vi "main 0.1.vi"() -> ()   [LabVIEW 2015]
uses:
  subvi/Newport ESP301/Newport ESP301.lvlib
  subvi/sp_manip.llb/sp_manip_lib.lvlib
  subvi/sp_manip.llb/tcp_gateway.lvlib
panel:
  out "error IO":errorcluster
  out "ESP_con?":bool caption="ESP301"
  out "phoib_con?":bool caption="PHOIBOS"
  out "manip_con?":bool caption="manipulator"
  out "cam_con?":bool caption="camera"
  in  "main_close":bool
  in  "Tab Control":enum32{"Live", "Measure", "Settings", "Devices"}(tab)
  out "Intensity Graph":u16[][](graph)
  out "Saved Positions":string[][](table)=[["ertwertwert", "-2.299945", "-2.030214", "38.900024", "50.000762", "0.000887", "-97.998082"], ["uztgugt", "-14.999451", "-13.638894", "442.380066", "13.998380", "-1.893758", "-76.305838"], ["asdf", "-14.999451", "-13.638894", "442.380066", "13.998380", "-1.893758", "-76.305838"], ["test3", "-14.999451", "-13.638894", "441.380066", "13.998380", "-1.893758", "-76.305838"]]
  in  "Save Pos":bool
  in  "Load":bool
  in  "Delete":bool
  in  "ManipRel":dbl=1.0
  in  "ManipRel +":bool
  in  "ManipRel -":bool
  in  "manip.rel.select":enum32{"x", "y", "z", "polar", "tilt", "azimut"}(radio)=enum."polar"
  in  "Move Abs":bool
  in  "stop manip":bool
  in  "dest":dbl[](array[numeric])=[0.007141549166819264, -0.009888298846365134, 431.30615234375, 89.00040512814502, 1.109125024699864, -227.9162918846475] caption="destinations" format="%#.5g"
  out "names":string[](array[string])=["x", "y", "z", "polar", "tilt", "azimut"]
  out "pos":dbl[](array[numeric])=[0.007141549166819264, -0.009888298846365134, 431.30615234375, 89.00040512814502, 1.109125024699864, -227.9162918846475] caption="positions" format="%.5f"
  in  "Delay":dbl format="%.1f"
  in  "Exposure":dbl=1000.0 format="%.1f"
  in  "Vertical binning":u16=4
  in  "Horzontal binning":u16=4
  in  "ROI Bottom":i32=33
  in  "ROI Top":i32=1
  in  "ROI Right":i32=43
  in  "ROI Left":i32=1
  out "opti_frames":dbl=25.0 caption="#steps_opti"
  out "opti_current_frame":i32=25
  out "Measurement Progress":u8(slide) scale=0.0..100.0
  out "Camera Aquisition":u8(slide) scale=0.0..100.0
  in  "Optimize":bool
  in  "OptiStepSize":dbl=-1.0 caption="Step Size"
  in  "OptiRange":dbl=25.0 caption="Range"
  in  "meas_axis":string(combo)="tilt" caption="Axis"
  in  "OptiFrameAcc.":i32=60 caption="Frames2Average"
  in  "OptiCancel":bool
  out "#steps_opti":dbl=25.0
  out "current_step_opti":i32=25
  out "ETA":string
  in  "BasePath":path=path "Z:/PESdata"
  in  "Path":path=path "Z:/software/ManipulatorControl/save.txt"
  in  "ESP301 VISA":refnum<visa-resource-name>
  in  "cam_boardnr":i32
  # "step _ of _"
  # "step _ of _"
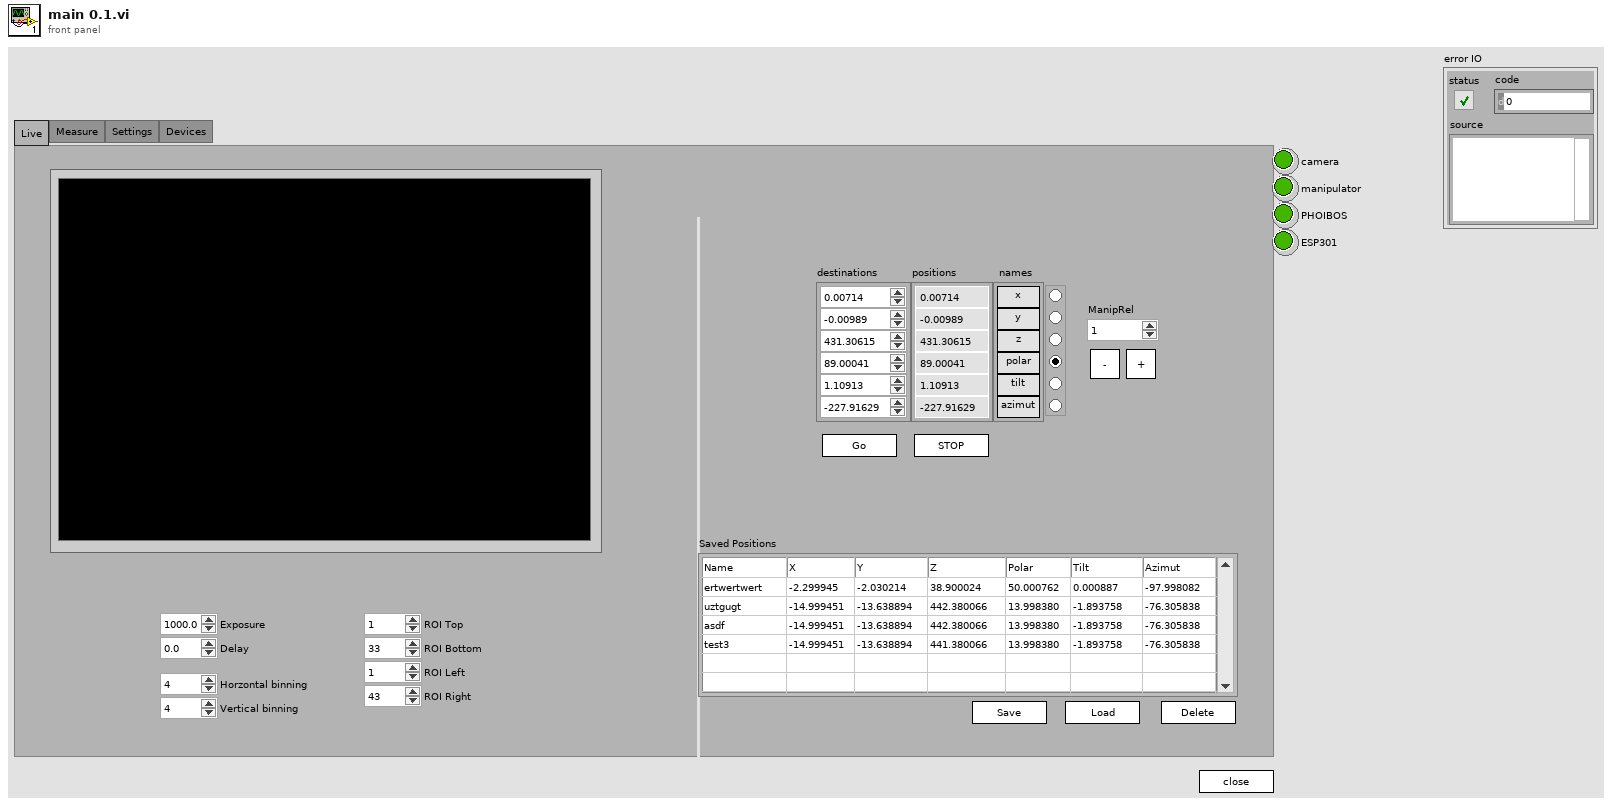
[diagram p1: front panel]
types:
  T1 = cluster{"Camera type":u32, "Operating mode\nHP & QE / HS & DiCam Pro ":u32, "Frame trigger \n(High Performance and QE only)":u16, "Sequence trigger":u16, "Low Light\n(QE only)":bool, "Gain":bool, "Horzontal\nbinning":u16, "Vertical\nbinning ":u16, "ROI Left":i32, "ROI Right":i32, "ROI Top":i32, "ROI Bottom":i32}
  T2 = cluster{"Axis_Name":string, "Axis_Type":string, "Axis_Position":dbl, "continous":bool, "moving":bool}[]
  T3 = cluster{"Axis_Name":string, "Axis_Type":string, "Axis_Position":dbl, "continous":bool, "moving":bool}
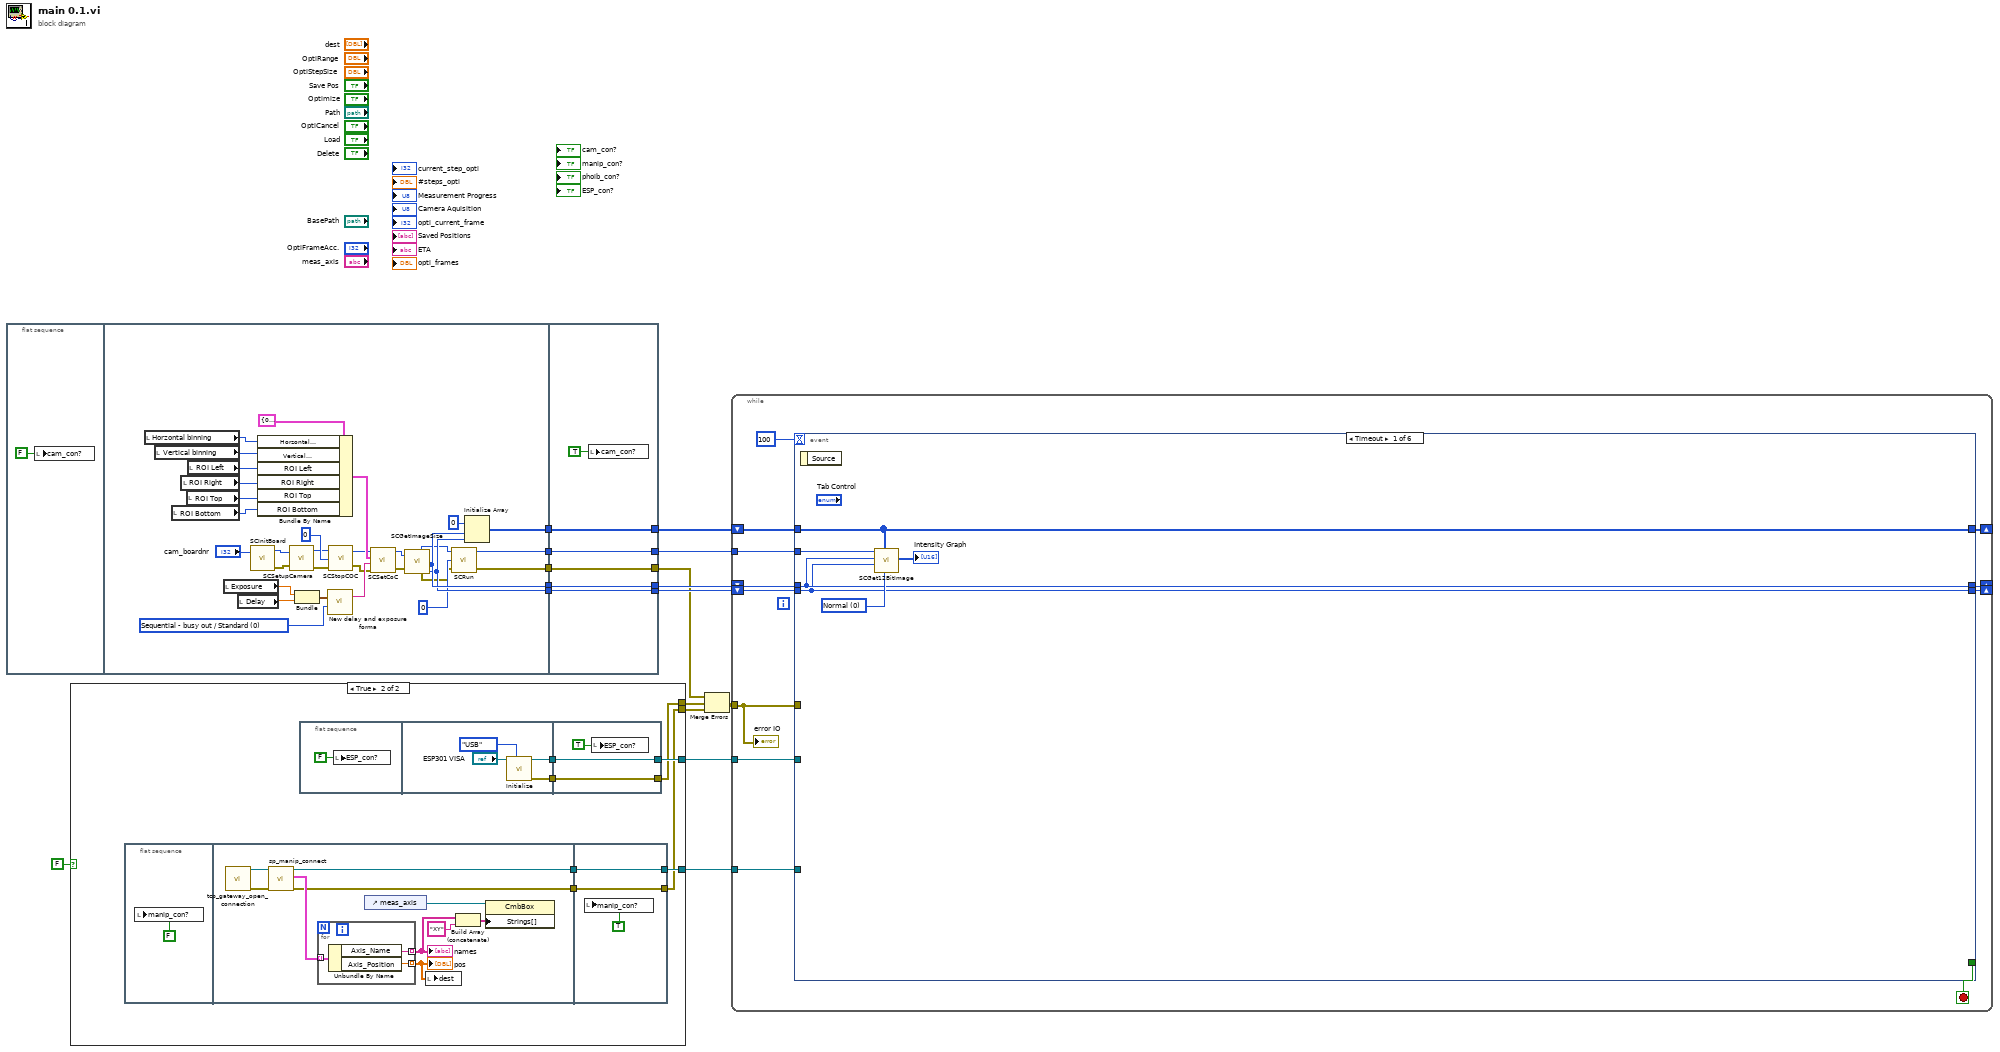
[diagram p0: block diagram]
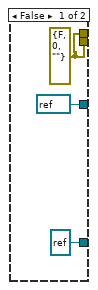
[diagram p2: hidden frame]
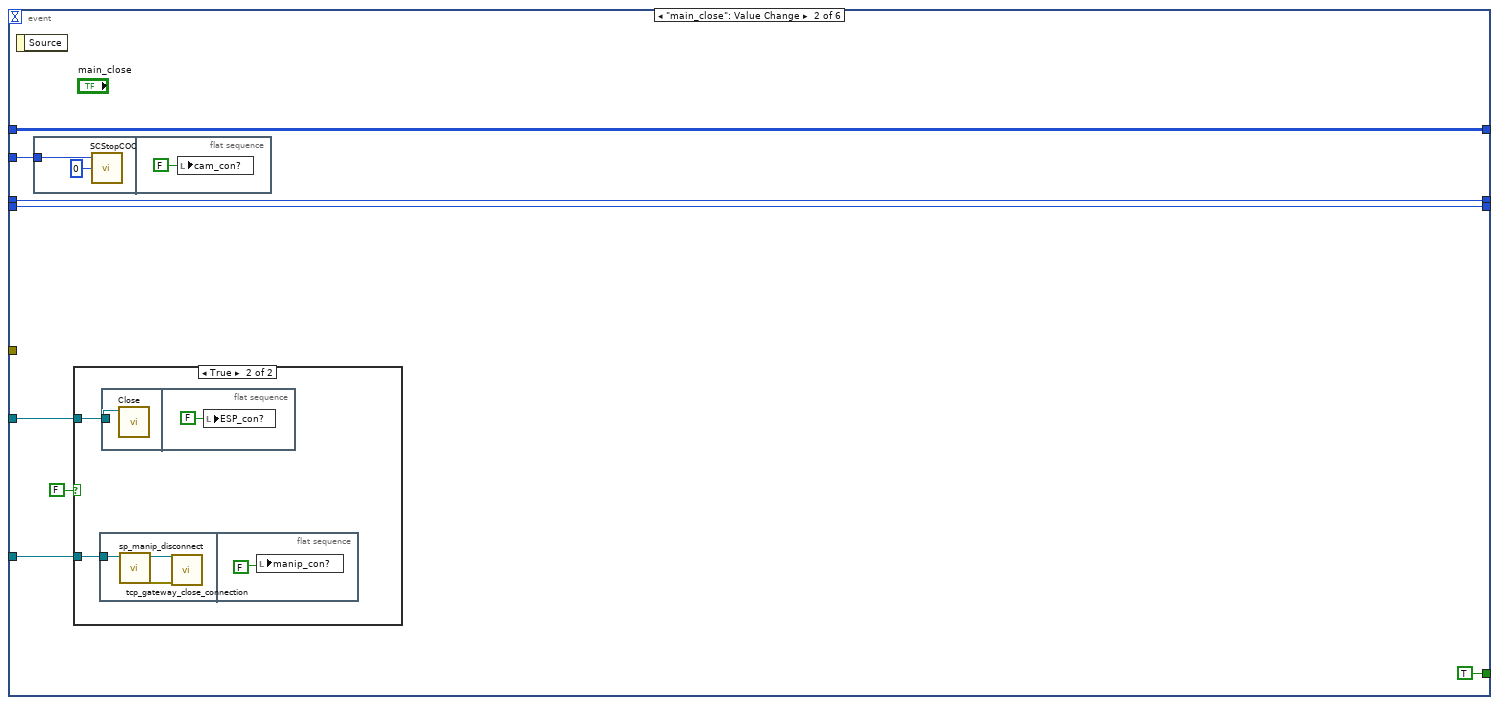
[diagram p3: hidden frame]
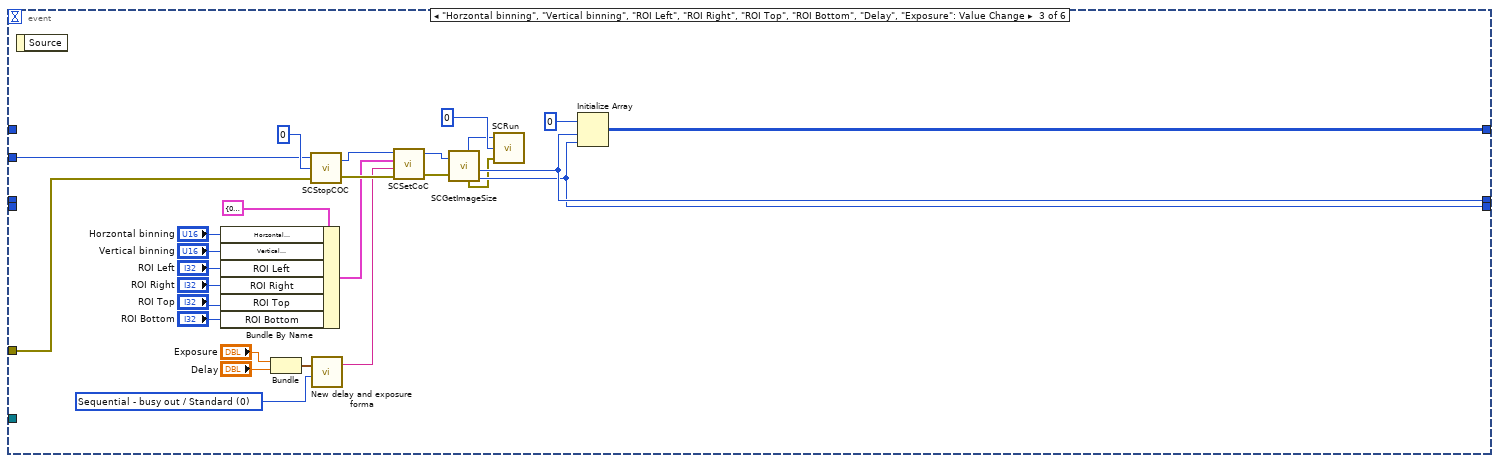
[diagram p5: hidden frame]
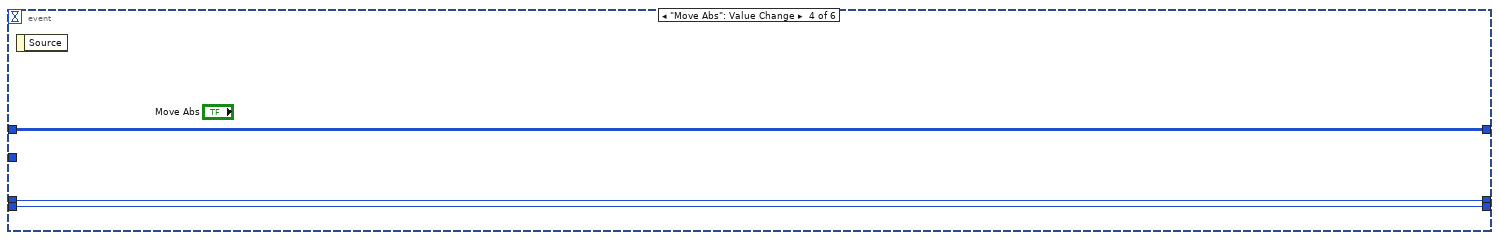
[diagram p6: hidden frame]
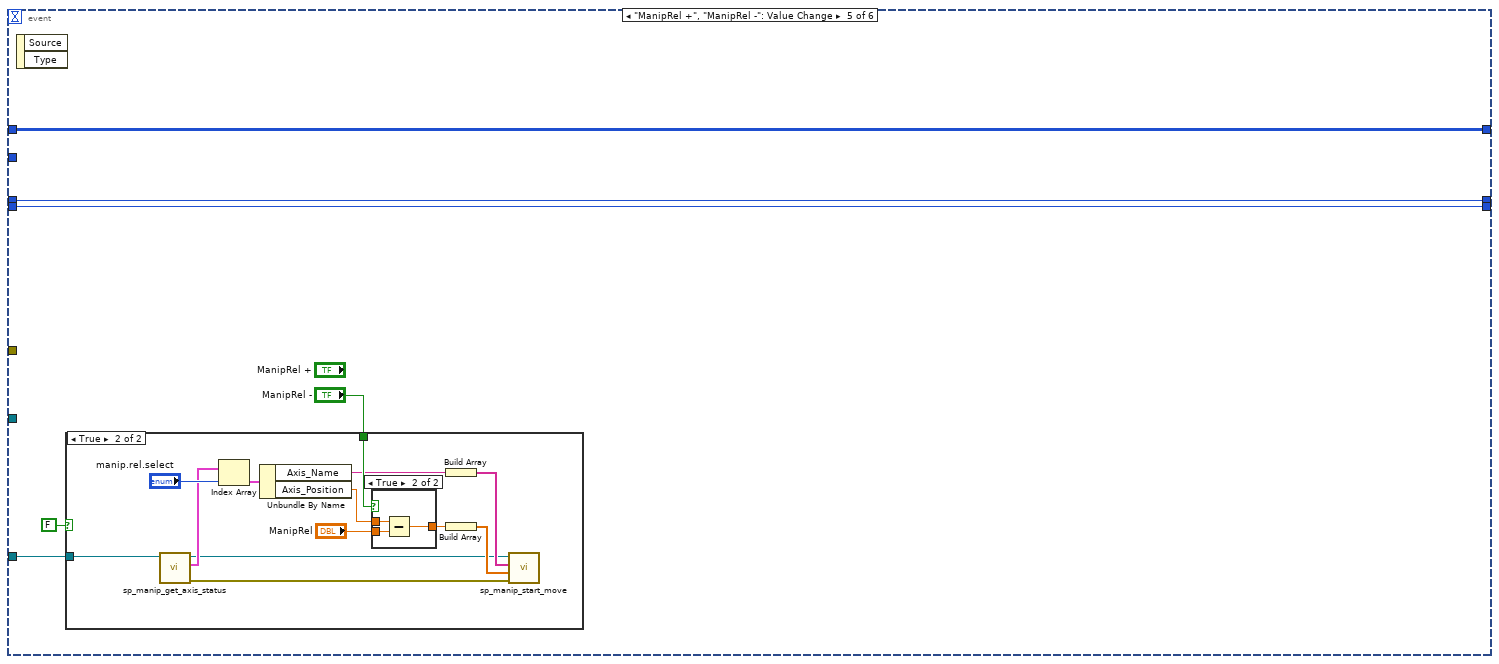
[diagram p7: hidden frame]
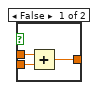
[diagram p9: hidden frame]
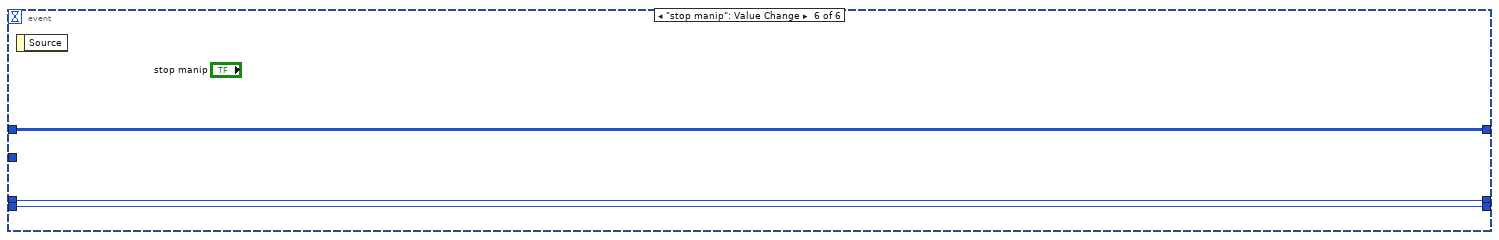
[diagram p10: hidden frame]
diagram:
  n1 = flat-sequence {
    tunnel: [w42] -> w6
    tunnel: [w38] -> w5
    tunnel: [w37] -> w4
    tunnel: [w28] -> w3
    tunnel: [w27] -> w2
    tunnel: [w51] -> w7
    tunnel: [w52] -> w8
    tunnel: [w53] -> w9
    tunnel: [w54] -> w10
    tunnel: [w55] -> w11
    tunnel: w6 -> [w55]
    tunnel: w5 -> [w54]
    tunnel: w4 -> [w53]
    tunnel: w3 -> [w52]
    tunnel: w2 -> [w51]
    frame #0 {
      n2 = local write "cam_con?"(FALSE ("cam_con?")) -> ()
    }
    frame #1 {
      w26 = u32 0 items=["Sequential - busy out / Standard"=0, "Simultaneous - busy out / 200 ns Double shot"=1, "Sequential - exposure out / 1000 ns Double shot"=2, "Simultaneous - exposure out / Reserved"=3, "Fast Frame / Fast cycle"=5, "QE short exposure"=8, "QE double shot"=9] ("Operating mode\nHP & QE / HS & DiCam Pro")
      n3 = local read "Horzontal binning"() -> (w36:u16)
      n4 = local read "Vertical binning"() -> (w35:u16)
      n5 = local read "ROI Bottom"() -> (w31:i32)
      n6 = local read "ROI Right"() -> (w33:i32)
      n7 = local read "ROI Top"() -> (w32:i32)
      n8 = local read "ROI Left"() -> (w34:i32)
      n9 = local read "Exposure"() -> (w25:dbl)
      n10 = local read "Delay"() -> (w24:dbl)
      n11 = call "SCInitBoard.vi"("boardnr"="cam_boardnr") -> ("Hout"=w47:u32, "error out"=w46:errorcluster)  [unwired: 1 in, 1 out]
      n12 = Bundle By Name(cluster=T1 {"Camera type"=0, "Operating mode\nHP & QE / HS & DiCam Pro "=0, "Frame trigger \n(High Performance and QE only)"=0, "Sequence trigger"=0, "Low Light\n(QE only)"=FALSE, "Gain"=FALSE, "Horzontal\nbinning"=0, "Vertical\nbinning "=0, "ROI Left"=1, "ROI Right"=20, "ROI Top"=1, "ROI Bottom"=15} ("Camera controls"), "Horzontal\nbinning"=w36, "Vertical\nbinning"=w35, "ROI Left"=w34, "ROI Right"=w33, "ROI Top"=w32, "ROI Bottom"=w31) -> (w40:T1)
      n13 = call "SCSetupCamera.vi"("Handle"=w47, "error in (no error)"=w46) -> ("Hout"=w45:u64, "error out"=w44:errorcluster)  [unwired: 1 out]
      n14 = Bundle("Exposure"=w25, "Delay"=w24) -> (w39:cluster{"Exposure ":dbl, "Delay":dbl})  [unwired: 1 in]
      n15 = call "New delay and exposure forma.vi"("Operating mode\nHP & QE / HS & DiCam Pro"=w26, "Delay and exposure"=w39) -> ("Output table"=w30:string)  [unwired: 3 in]
      n16 = call "SCStopCOC.vi"("error in (no error)"=w44, "Stop mode"=0, "Handle"=w45) -> ("error out"=w23:errorcluster, "Hout"=w22:u64)
      n17 = call "SCSetCoC.vi"("error in (no error)"=w23, "Delay and exposure table"=w30, "Camera controls"=w40, "Handle"=w22) -> ("error out"=w20:errorcluster, "Hout"=w21:u64)  [unwired: 1 out]
      n18 = call "SCGetImageSize.vi"("Handle"=w21, "error in (no error)"=w20) -> ("Hout"=w19:u64, "error out"=w18:errorcluster, "Horizontal size"=w38:i32, "Vertical size"=w37:i32)  [unwired: 2 out]
      n19 = call "SCRun.vi"("error in (no error)"=w18, "Run mode"=0, "Handle"=w19) -> ("error out"=w27:errorcluster, "Run error out"=w28:i32)  [unwired: 1 out]
      n20 = Initialize Array(u16 0 ("dimension size"), w38, w37) -> (w42:u16[][])
    }
    frame #2 {
      n21 = local write "cam_con?"(TRUE ("cam_con?")) -> ()
    }
  }
  n22 = case shown="True" FALSE {
    tunnel: [refnum<visa-resource-name> refnum ("VISA resource name out") w62] -> w16
    tunnel: [refnum<k5> refnum ("gateway_connection out") w61] -> w15
    tunnel: [w56 w60] -> w14
    tunnel: [w56 w59] -> w13
    frame False {
      w56 = errorcluster {"status"=FALSE, "code"=0, "source"=""} ("error out")
    }
    frame True {
      n23 = flat-sequence {
        tunnel: [w77] -> w66
        tunnel: [w85] -> w65
        tunnel: [w90] -> w61
        tunnel: [w91] -> w60
        tunnel: w66 -> [w91]
        tunnel: w65 -> [w90]
        frame #0 {
          n24 = local write "manip_con?"(FALSE ("manip_con?")) -> ()
        }
        frame #1 {
          n25 = call "tcp_gateway_open_connection.vi"() -> ("gateway_connection"=w80:refnum<k5>, "error out"=w79:errorcluster)  [unwired: 5 in, 3 out]
          n26 = call "sp_manip_connect.vi"("error in"=w79, "gateway_connection"=w80) -> ("error out"=w77:errorcluster, "axis_out"=w78:T2, "gateway_connection out"=w85:refnum<k5>)  [unwired: 5 in, 2 out]
          n27 = for {
            tunnel: w78 -> [w88] mode=indexing
            tunnel: [w87] -> w83 mode=indexing
            tunnel: [w86] -> w84 mode=indexing
            n28 = Unbundle By Name(w88) -> ("Axis_Name"=w87:string, "Axis_Position"=w86:dbl)
          }
          "names" <- w83
          "pos" <- w84
          n29 = control-ref of="meas_axis"() -> (w76:refnum<vi>)
          n30 = local write "dest"(w84) -> ()
          n31 = Build Array (concatenate)(w83, "XY") -> (w81:string[])
          n32 = property on="Property Node" class="CmbBox"(reference=w76, "Strings[]"=w81) -> ()  [unwired: 1 in, 2 out]
        }
        frame #2 {
          n33 = local write "manip_con?"(TRUE ("manip_con?")) -> ()
        }
      }
      n34 = flat-sequence {
        tunnel: [w69] -> w64
        tunnel: [w68] -> w63
        tunnel: [w73] -> w59
        tunnel: [w74] -> w62
        tunnel: w64 -> [w74]
        tunnel: w63 -> [w73]
        frame #0 {
          n35 = local write "ESP_con?"(FALSE ("manip_con?")) -> ()
        }
        frame #1 {
          n36 = call "Initialize.vi"("VISA resource name"="ESP301 VISA", "Serial Link (RS232)"=enum16{"RS232", "USB"}."USB") -> ("VISA resource name out"=w69:refnum<visa-resource-name>, "error out"=w68:errorcluster)  [unwired: 7 in]
        }
        frame #2 {
          n37 = local write "ESP_con?"(TRUE ("manip_con?")) -> ()
        }
      }
    }
  }
  n38 = Merge Errors(w7, w13, w14) -> (w12:errorcluster)
  n39 = while {
    tunnel: w16 -> [w102]
    tunnel: w12 -> [w101]
    tunnel: w15 -> [w100]
    tunnel: w8 -> [w98]
    shift-right: [w94] -> _
    shift-left: w10 -> [w97]
    shift-right: [w93] -> _
    shift-left: w9 -> [w96]
    shift-right: [w92] -> _
    shift-left: w11 -> [w99]
    stop <- w103 stop-if-true
    n40 = event shown="[0] Timeout" {
      selector: _ -> [_ _ _ _ _ _]
      dyn-events: _ -> [_ _ _ _ _ _]
      timeout: 100 -> [_ _ _ _ _ _]
      tunnel: [_ TRUE _ _ _ _] -> w103
      tunnel: w102 -> [_ w116 _ _ _ _]
      tunnel: w101 -> [_ _ w137 _ _ _]
      tunnel: w100 -> [_ w115 _ _ w164 _]
      tunnel: w99 -> [w104 w112 _ w156 w161 w186]
      tunnel: w98 -> [w108 w114 w138 _ _ _]
      tunnel: w97 -> [w106 w111 _ w157 w160 w185]
      tunnel: w96 -> [w105 w110 _ w158 w159 w184]
      tunnel: [w106 w111 w135 w157 w160 w185] -> w94
      tunnel: [w105 w110 w134 w158 w159 w184] -> w93
      tunnel: [w104 w112 w133 w156 w161 w186] -> w92
      event Timeout {
        w107 = 0 items=["Normal", "Upside down"] ("mode")
        n41 = event-data() -> ()  [unwired: 1 in, 1 out]
        n42 = call "SCGet12BitImage.vi"("mode"=w107, "Input array"=w104, "Vertical size"=w105, "Horizontal size"=w106, "Handle"=w108) -> ("imgdata"=→"Intensity Graph":u16[][])  [unwired: 2 in, 2 out]
      }
      event "main_close": Value Change {
        n43 = event-data() -> ()  [unwired: 1 in, 1 out]
        n44 = flat-sequence {
          tunnel: w114 -> [w127]
          frame #0 {
            n45 = call "SCStopCOC.vi"("Stop mode"=0, "Handle"=w127) -> ()  [unwired: 1 in, 2 out]
          }
          frame #1 {
            n46 = local write "cam_con?"(FALSE ("cam_con?")) -> ()
          }
        }
        n47 = case shown="True" FALSE {
          tunnel: w116 -> [_ w119]
          tunnel: w115 -> [_ w118]
          frame False {
          }
          frame True {
            n48 = flat-sequence {
              tunnel: w118 -> [w120]
              frame #0 {
                n49 = call "sp_manip_disconnect.vi"("gateway_connection"=w120) -> ("error out"=w121:errorcluster, "gateway_connection_out"=w122:refnum<k5>)  [unwired: 7 in, 2 out]
                n50 = call "tcp_gateway_close_connection.vi"("error in"=w121, "server_connection"=w122) -> ()  [unwired: 5 in, 1 out]
              }
              frame #1 {
                n51 = local write "manip_con?"(FALSE ("manip_con?")) -> ()
              }
            }
            n52 = flat-sequence {
              tunnel: w119 -> [w124]
              frame #0 {
                n53 = call "Close.vi"("VISA resource name"=w124) -> ()  [unwired: 10 in, 1 out]
              }
              frame #1 {
                n54 = local write "ESP_con?"(FALSE ("manip_con?")) -> ()
              }
            }
          }
        }
      }
      event "Horzontal binning", "Vertical binning", "ROI Left", "ROI Right", "ROI Top", "ROI Bottom", "Delay", "Exposure": Value Change {
        w147 = u32 0 items=["Sequential - busy out / Standard"=0, "Simultaneous - busy out / 200 ns Double shot"=1, "Sequential - exposure out / 1000 ns Double shot"=2, "Simultaneous - exposure out / Reserved"=3, "Fast Frame / Fast cycle"=5, "QE short exposure"=8, "QE double shot"=9] ("Operating mode\nHP & QE / HS & DiCam Pro")
        n55 = event-data() -> ()  [unwired: 1 in, 1 out]
        n56 = Bundle By Name(cluster=T1 {"Camera type"=0, "Operating mode\nHP & QE / HS & DiCam Pro "=0, "Frame trigger \n(High Performance and QE only)"=0, "Sequence trigger"=0, "Low Light\n(QE only)"=FALSE, "Gain"=FALSE, "Horzontal\nbinning"=0, "Vertical\nbinning "=0, "ROI Left"=1, "ROI Right"=20, "ROI Top"=1, "ROI Bottom"=15} ("Camera controls"), "Horzontal\nbinning"="Horzontal binning", "Vertical\nbinning"="Vertical binning", "ROI Left"="ROI Left", "ROI Right"="ROI Right", "ROI Top"="ROI Top", "ROI Bottom"="ROI Bottom") -> (w150:T1)
        n57 = Bundle("Exposure"="Exposure", "Delay"="Delay") -> (w148:cluster{"Exposure ":dbl, "Delay":dbl})  [unwired: 1 in]
        n58 = call "SCStopCOC.vi"("error in (no error)"=w137, "Stop mode"=0, "Handle"=w138) -> ("error out"=w155:errorcluster, "Hout"=w154:u64)
        n59 = call "New delay and exposure forma.vi"("Operating mode\nHP & QE / HS & DiCam Pro"=w147, "Delay and exposure"=w148) -> ("Output table"=w151:string)  [unwired: 3 in]
        n60 = call "SCSetCoC.vi"("error in (no error)"=w155, "Delay and exposure table"=w151, "Camera controls"=w150, "Handle"=w154) -> ("error out"=w132:errorcluster, "Hout"=w131:u64)  [unwired: 1 out]
        n61 = call "SCGetImageSize.vi"("Handle"=w131, "error in (no error)"=w132) -> ("Hout"=w130:u64, "error out"=w129:errorcluster, "Horizontal size"=w135:i32, "Vertical size"=w134:i32)  [unwired: 2 out]
        n62 = call "SCRun.vi"("error in (no error)"=w129, "Run mode"=0, "Handle"=w130) -> ()  [unwired: 3 out]
        n63 = Initialize Array(u16 0 ("dimension size"), w135, w134) -> (w133:u16[][])
      }
      event "Move Abs": Value Change {
        n64 = event-data() -> ()  [unwired: 1 in, 1 out]
      }
      event "ManipRel +", "ManipRel -": Value Change {
        n65 = event-data() -> ()  [unwired: 1 in, 2 out]
        n66 = case shown="True" FALSE {
          tunnel: w164 -> [_ w176]
          tunnel: "ManipRel -" -> [_ w173]
          frame False {
          }
          frame True {
            n67 = call "sp_manip_get_axis_status.vi"("gateway_connection"=w176) -> ("error out"=w169:errorcluster, "axis_out"=w175:T2, "gateway_connection out"=w165:refnum<k5>)  [unwired: 6 in, 2 out]
            n68 = Index Array(array=w175, index="manip.rel.select") -> (element=w174:T3)
            n69 = Unbundle By Name(w174) -> ("Axis_Name"=w166:string, "Axis_Position"=w168:dbl)
            n70 = case shown="True" w173 {
              tunnel: [w180 w183] -> w172
              tunnel: w168 -> [w179 w182]
              tunnel: "ManipRel" -> [w178 w181]
              frame False {
                n71 = Add(x=w179, y=w178) -> (x+y=w180:dbl)
              }
              frame True {
                n72 = Subtract(x=w182, y=w181) -> (x-y=w183:dbl)
              }
            }
            n73 = Build Array(w166) -> (w171:string[])
            n74 = Build Array(w172) -> (w170:dbl[])
            n75 = call "sp_manip_start_move.vi"("error in"=w169, "target positions"=w170, "axis names"=w171, "gateway_connection"=w165) -> ()  [unwired: 4 in, 4 out]
          }
        }
      }
      event "stop manip": Value Change {
        n76 = event-data() -> ()  [unwired: 1 in, 1 out]
      }
    }
    "error IO" <- w101
  }
